vi "Stellungen_Namen2.vi"(0 "Kühlventil":dbl(slide) scale=0.02..0.004, 4 "Pumpensteuerung":dbl min=0.0 max=10.0 step=0.1, 5 "Regelventil 39":dbl(slide) scale=0.02..0.004, 6 "Exp.V":dbl(slide) min=0.0 max=10.0 step=1e-05 scale=0.0..10.0, 7 "Regelventil 14":dbl(slide) scale=0.02..0.004, 8 "Meter":dbl(knob) min=0.0 max=1500.0 scale=0.0..1500.0, 9 "zu":bool, 10 "auf":bool, 11 "Regelventil 35":dbl(slide) scale=0.02..0.004) -> (3 "Dynamic Data":dynamicdata(waveform))   [LabVIEW 2015]
uses:
  <vilib>/express/express shared/transition.llb/Dynamic To Waveform Array.vi
  <vilib>/express/express signal manip/GetorSetDDTAttributes/Set DDT Attributes/SetT0.vi
  <vilib>/express/express shared/transition.llb/Waveform Array To Dynamic.vi
  <vilib>/express/express signal manip/GetorSetDDTAttributes/Set DDT Attributes/Set DDT Properties.xnode
panel:
  in  "Verdichter Bestätigung":bool
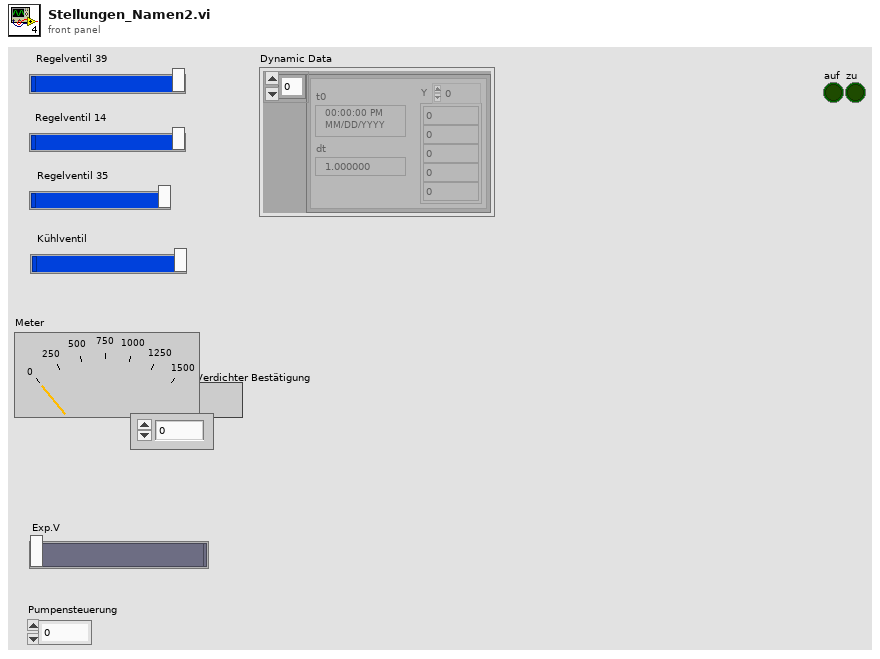
[diagram p1: front panel]
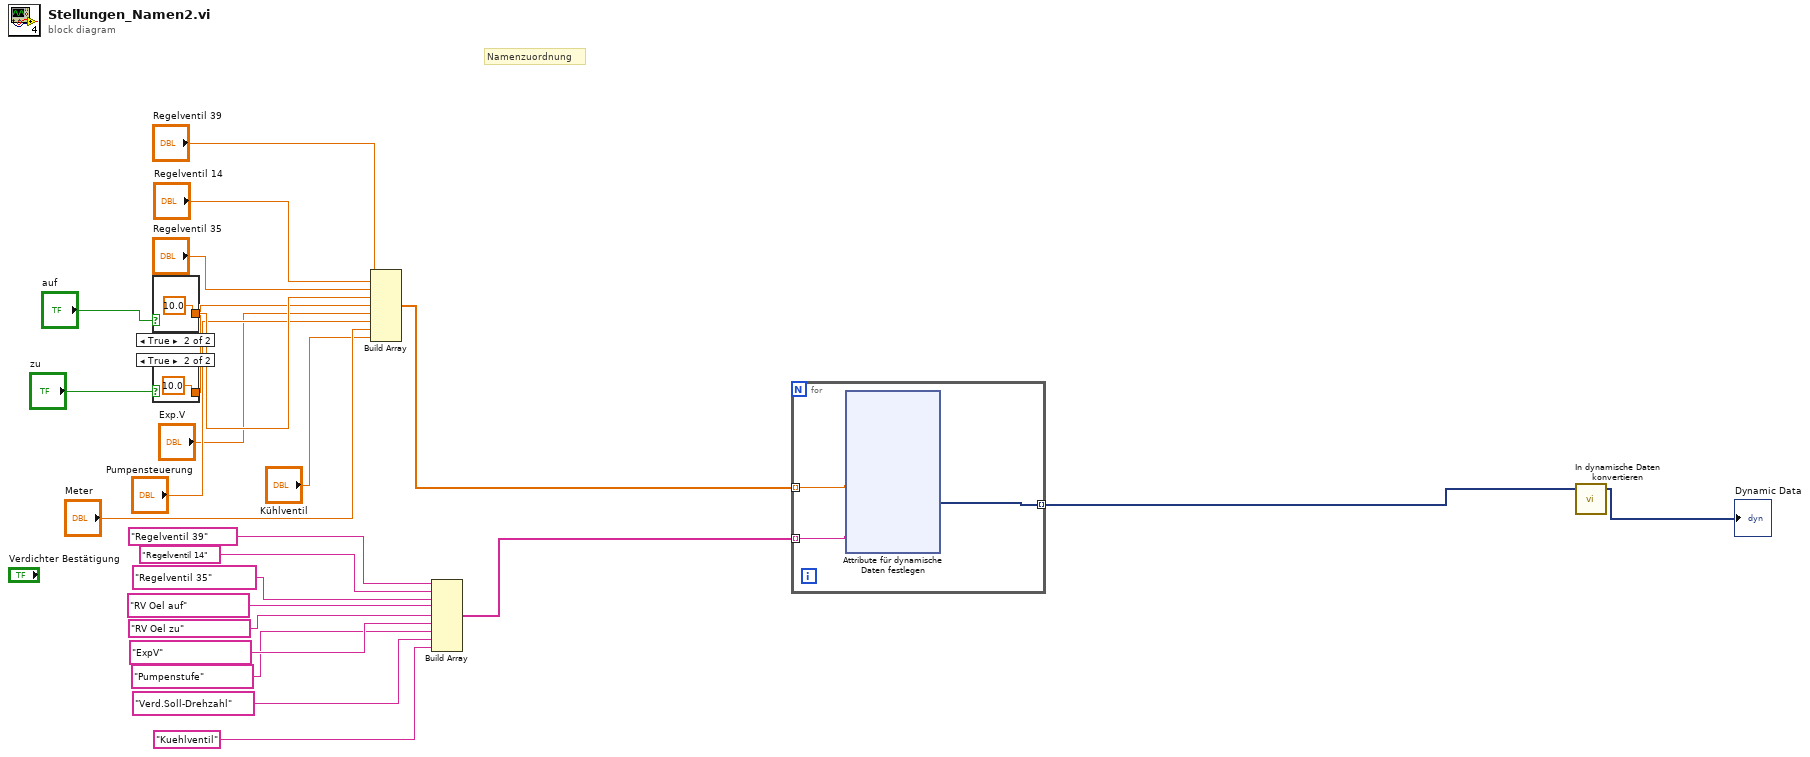
[diagram p0: block diagram]
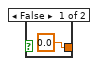
[diagram p2: hidden frame]
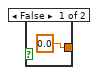
[diagram p3: hidden frame]
diagram:
  # "Namenzuordnung"
  n1 = case shown="True" "auf" {
    tunnel: [0.0 10.0] -> w16
    frame False {
    }
    frame True {
    }
  }
  n2 = case shown="True" "zu" {
    tunnel: [0.0 10.0] -> w15
    frame False {
    }
    frame True {
    }
  }
  n3 = Build Array("Regelventil 39", "Regelventil 14", "Regelventil 35", w16, w15, "Exp.V", "Pumpensteuerung", "Meter", "Kühlventil") -> (w22:dbl[])
  n4 = Build Array("Regelventil 39", "Regelventil 14", "Regelventil 35", "RV Oel auf", "RV Oel zu", "ExpV", "Pumpenstufe", "Verd.Soll-Drehzahl", "Kuehlventil" ("element")) -> (w23:string[])
  n5 = for {
    tunnel: [w31] -> w13 mode=indexing
    tunnel: w23 -> [w30] mode=indexing
    tunnel: w22 -> [w29] mode=indexing
    n6 = xnode "Attribute für dynamische Daten festlegen"("Signals In"=w29, "Signal Name"=w30) -> ("Signals Out"=w31:dynamicdata)  [unwired: 2 in, 1 out]
  }
  n7 = call "In dynamische Daten konvertieren"("Array of Waveforms"=w13) -> ("Dynamic Data Type"=→"Dynamic Data":dynamicdata)  [unwired: 3 in]
